vi "sub_SDR_mimo_rx.vi"(6 "Init Rx Buffer":bool, 7 "System options":T1={"Samples per symbol"=6, "Roll-Off"=0.75, "Filter length (symbols)"=7, "Modulation Type"=enum."64-QAM", "Payload Symbols"=1472, "Symbols per Pilot"=6} {"Symbols per Pilot" min=6 max=16 step=2; "Payload Symbols" min=16 max=8192 step=16; "Filter length (symbols)" min=1 max=9 step=2; "Roll-Off" min=0.0 max=1.0 step=0.01; "Samples per symbol" min=2 max=32 step=2}, 10 "Radio Frame":cdb[][](array[numeric])) -> (0 "Constellation Data":cluster{dbl[], dbl[]}[](array[cluster]), 1 "Pilot SNR After equalization":dbl[](array[numeric]), 2 "SNR Before Equalizer":dbl[](array[numeric]), 3 "Received Packets in current frame":string[](array[string]), 4 "Received Data SNR":dbl[](array[numeric]))   [LabVIEW 2012]
panel:
  out "Packet Synch?":bool
  out "Last received packet num":i32
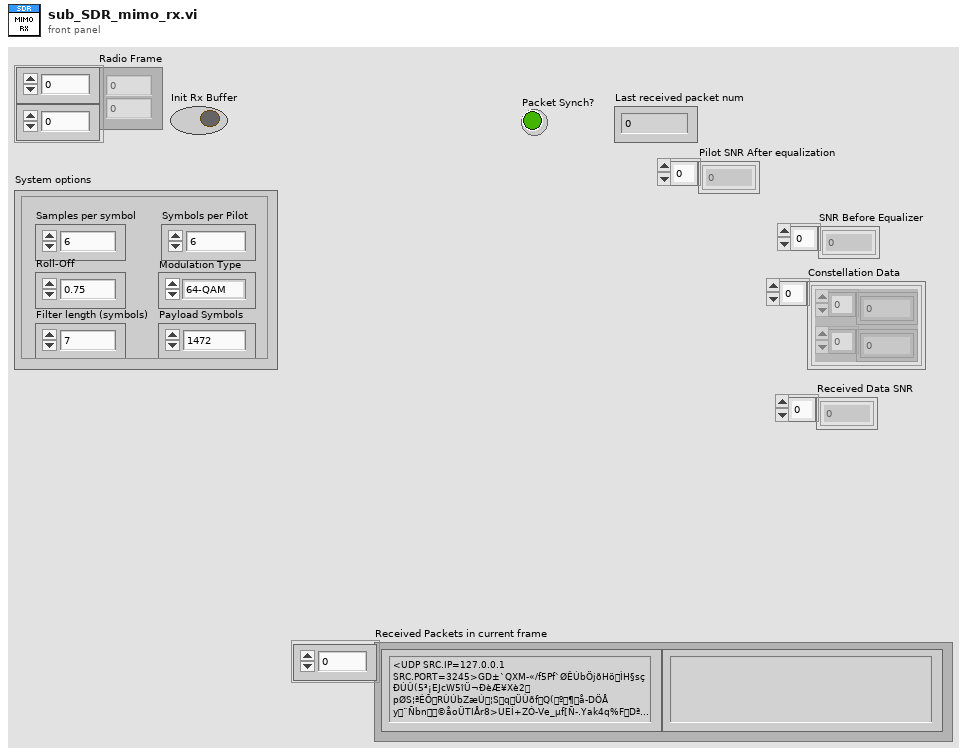
[diagram p1: front panel]
types:
  T1 = cluster{"Samples per symbol":i32, "Roll-Off":dbl, "Filter length (symbols)":i32, "Modulation Type":enum16{"BPSK", "4-QAM", "16-QAM", "64-QAM"}, "Payload Symbols":i32, "Symbols per Pilot":i32}
  T2 = cluster{"Samples per symbol":i32, "Roll-Off":dbl, "Filter length (symbols)":i32}
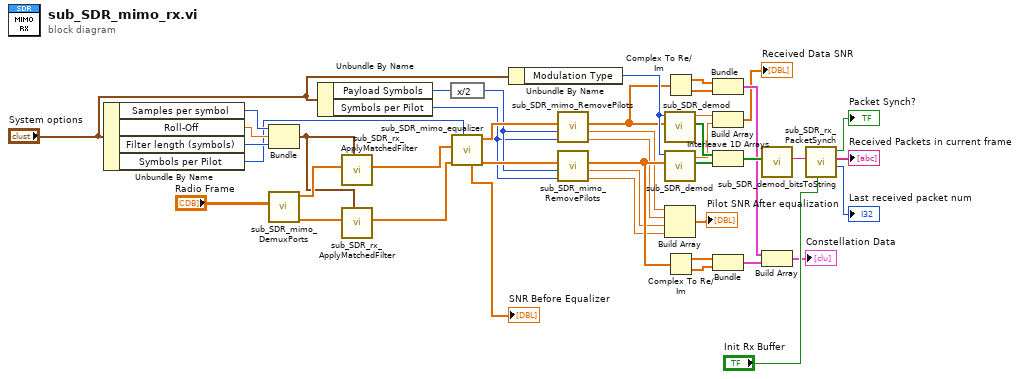
[diagram p0: block diagram]
diagram:
  n1 = Unbundle By Name("System options") -> ("Samples per symbol"=w23:i32, "Roll-Off"=w22:dbl, "Filter length (symbols)"=w21:i32, "Symbols per Pilot"=w16:i32)
  n2 = Bundle("Samples per symbol"=w23, "Roll-Off"=w22, "Filter length (symbols)"=w21) -> (w20:T2)  [unwired: 1 in]
  n3 = call "sub_SDR_mimo_DemuxPorts.vi"("Data in (2D)"="Radio Frame") -> ("Port 2"=w33:cdb[], "Port 1"=w32:cdb[])  [unwired: 9 in]
  n4 = Unbundle By Name("System options") -> ("Payload Symbols"=w19:i32, "Symbols per Pilot"=w15:i32)
  n5 = call "sub_SDR_rx_ApplyMatchedFilter.vi"("Filter Options"=w20, "Received stream"=w32) -> ("Received Symbols"=w30:cdb[])  [unwired: 9 in]
  n6 = call "sub_SDR_rx_ApplyMatchedFilter.vi"("Filter Options"=w20, "Received stream"=w33) -> ("Received Symbols"=w31:cdb[])  [unwired: 9 in]
  n7 = expression code="x/2"(w19) -> (w18:i32)
  n8 = call "sub_SDR_mimo_equalizer.vi"("Symbols per Pilot"=w16, "Input Symbols Port 2"=w31, "Input Symbols Port 1"=w30) -> ("Output symbols Port 2"=w35:cdb[], "Output symbols Port 1"=w34:cdb[], "SNR Before Equalizer"=→"SNR Before Equalizer":dbl[])  [unwired: 6 in]
  n9 = Unbundle By Name("System options") -> ("Modulation Type"=w36:enum16{"BPSK", "4-QAM", "16-QAM", "64-QAM"})
  n10 = call "sub_SDR_mimo_RemovePilots.vi"("Symbols per pilot"=w15, "Payload Symbols"=w18, "Array in"=w34) -> ("SNR 2 (dB)"=w4:dbl, "SNR 1 (dB)"=w5:dbl, "Array Out"=w13:cdb[])  [unwired: 6 in]
  n11 = call "sub_SDR_mimo_RemovePilots.vi"("Symbols per pilot"=w15, "Payload Symbols"=w18, "Array in"=w35) -> ("SNR 2 (dB)"=w2:dbl, "SNR 1 (dB)"=w3:dbl, "Array Out"=w12:cdb[])  [unwired: 6 in]
  n12 = call "sub_SDR_demod.vi"("Input Symbols"=w13, "Modulation Type"=w36) -> ("Output bits"=w38:bool[], "SNR [dB]"=w9:dbl)  [unwired: 8 in]
  n13 = call "sub_SDR_demod.vi"("Input Symbols"=w12, "Modulation Type"=w36) -> ("Output bits"=w37:bool[], "SNR [dB]"=w8:dbl)  [unwired: 8 in]
  n14 = Build Array(w5, w4, w3, w2) -> (→"Pilot SNR After equalization":dbl[])
  n15 = Complex To Re/Im(x + iy=w13) -> (x=w24:dbl[], y=w25:dbl[])
  n16 = Complex To Re/Im(x + iy=w12) -> (x=w27:dbl[], y=w28:dbl[])
  n17 = Bundle(w24, w25) -> (w26:cluster{dbl[], dbl[]})  [unwired: 1 in]
  n18 = Build Array(w9, w8) -> (→"Received Data SNR":dbl[])
  n19 = Interleave 1D Arrays(w38, w37) -> (w39:bool[])
  n20 = Bundle(w27, w28) -> (w29:cluster{dbl[], dbl[]})  [unwired: 1 in]
  n21 = call "sub_SDR_demod_bitsToString.vi"("Input bits"=w39) -> ("Output string"=w41:string)  [unwired: 10 in]
  n22 = Build Array(w26, w29) -> (→"Constellation Data":cluster{dbl[], dbl[]}[])
  n23 = call "sub_SDR_rx_PacketSynch.vi"("Init?"="Init Rx Buffer", "Input Stream"=w41) -> ("Last received packet num"=→"Last received packet num":i32, "Output Packets"=→"Received Packets in current frame":string[], "Packet Synch?"=→"Packet Synch?":bool)  [unwired: 7 in]
